vi "Do.vi"(8 "error in (no error)":errorcluster, 10 "Actor in":refnum<class "Actor.lvclass">, 11 "Add LVProject Msg in":refnum<class "Add LVProject Msg.lvclass">) -> (0 "error out":errorcluster, 2 "Actor out":refnum<class "Actor.lvclass">)   [LabVIEW 2017, in "BuildServer.lvlib" / "Add LVProject Msg.lvclass"]
uses:
  Add LVProject Msg.lvclass
  <vilib>/ActorFramework/Actor/Actor.lvclass
  BuildServer/BuildServer.lvclass
  C:/Program Files (x86)/National Instruments/LabVIEW 2017/vi.lib/ActorFramework/Actor/Actor.lvclass
  Add LVProject Msg.lvclass/Add LVProject Msg.ctl
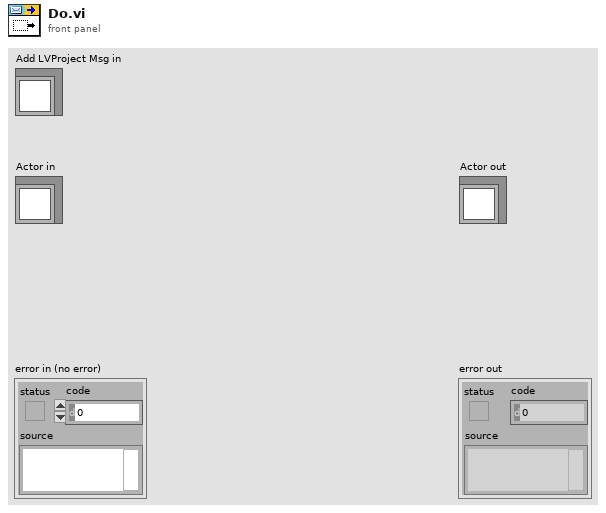
[diagram p1: front panel]
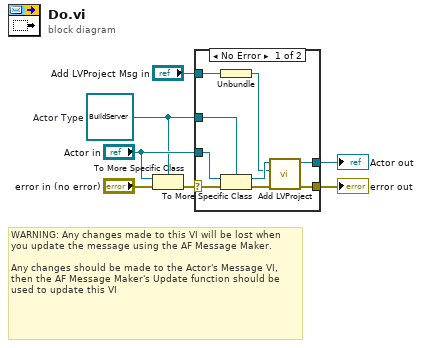
[diagram p0: block diagram]
diagram:
  w2 = refnum<class "BuildServer.lvclass"> refnum  # Actor Type
  # "WARNING: Any changes made to this VI will be lost when you update the message using the AF Message Maker.\n\nAny changes should be made to the Actor's Message VI, then the AF Message Maker's Update function should be used to update this VI"
  n1 = To More Specific Class(target class=w2, reference="Actor in", error in="error in (no error)") -> (error out=w6:errorcluster)  [unwired: 1 out]
  n2 = case shown="No Error" w6 {
    selector: w6 -> [w16 w18]
    tunnel: [w11 w18] -> w5
    tunnel: [w10 w17] -> w4
    tunnel: "Actor in" -> [w15 w17]
    tunnel: w2 -> [w14 _]
    tunnel: "Add LVProject Msg in" -> [w9 _]
    frame No Error {
      n3 = Unbundle(w9) -> (w8:path)
      n4 = To More Specific Class ("Actor Cast")(target class=w14, reference=w15, error in=w16) -> (specific class reference=w13:refnum<class "BuildServer.lvclass">, error out=w12:errorcluster)
      n5 = call "Add LVProject.vi"("error in (no error)"=w12, "Project Path"=w8, "BuildServer in"=w13) -> ("error out"=w11:errorcluster, "BuildServer out"=w10:refnum<class "BuildServer.lvclass">)  [unwired: 7 in]
    }
    frame Error {
    }
  }
  "error out" <- w5
  "Actor out" <- w4
